vi "name2time.vi"(4 "error in":errorcluster, 6 "f_name":string) -> (0 "error IO":errorcluster, 1 "m_pt":i32, 2 "time stamp":timestamp)   [LabVIEW 2010]
uses:
  <vilib>/Utility/miscctls.llb/LVDateTimeRec.ctl
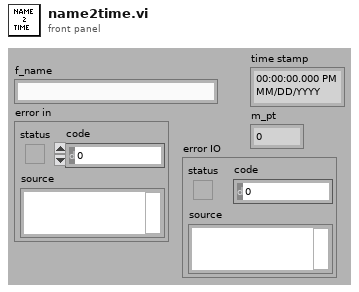
[diagram p1: front panel]
types:
  T1 = typedef "LVDateTimeRec.ctl" = cluster{"fractional second":dbl, "second":i32, "minute":i32, "hour":i32, "day of month":i32, "month":i32, "year":i32, "day of week":i32, "day of year":i32, "DST":i32}
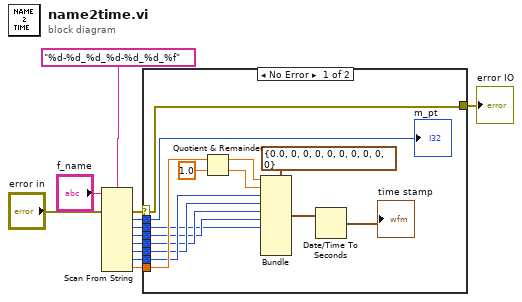
[diagram p0: block diagram]
diagram:
  n1 = Scan From String(format string="%d-%d_%d_%d-%d_%d_%f", input string="f_name", error in="error in") -> (error out=w2:errorcluster, output 1=w3:i32, output 2=w4:i32, output 3=w5:i32, output 4=w6:i32, output 5=w7:i32, output 6=w8:i32, output 7=w9:dbl)  [unwired: 8 in, 2 out]
  n2 = case shown="No Error" w2 {
    selector: w2 -> [w13 w27]
    tunnel: w9 -> [w24 _]
    tunnel: w8 -> [w20 _]
    tunnel: w7 -> [w19 _]
    tunnel: w6 -> [w18 _]
    tunnel: w5 -> [w17 _]
    tunnel: w4 -> [w16 _]
    tunnel: w3 -> [w15 _]
    tunnel: [w13 w27] -> w1
    frame No Error {
      n3 = Quotient & Remainder(x=w24, y=1.0) -> (x-y*floor(x/y)=w21:dbl, floor(x/y)=w22:dbl)
      n4 = Bundle(cluster=T1 {"fractional second"=0.0, "second"=0, "minute"=0, "hour"=0, "day of month"=0, "month"=0, "year"=0, "day of week"=0, "day of year"=0, "DST"=0} ("date time rec"), "fractional second"=w21, "second"=w22, "minute"=w20, "hour"=w19, "day of month"=w18, "month"=w17, "year"=w16) -> (w26:T1)  [unwired: 3 in]
      n5 = Date/Time To Seconds(2:w26) -> (0:→"time stamp":timestamp)  [unwired: 1 in]
      "m_pt" <- w15
    }
    frame Error {
    }
  }
  "error IO" <- w1
